vi "Configure Sweep Stimulus.vi"(4 "Signal Output (T: On)":bool=TRUE, 6 "Parameter (0.0)":dbl format="%^.2e", 7 "Channel (1)":i32=1, 8 "error in (no error)":errorcluster, 9 "Stimulus (0: Start)":u16(ring) items=["Start", "Stop", "Center", "Span"], 10 "Unit (0: Hz)":u16(ring) items=["Hz", "kHz", "MHz", "GHz", "dBm", "s", "V"], 11 "VISA resource name":refnum<visa-resource-name>) -> (0 "error out":errorcluster, 3 "VISA resource name out":refnum<visa-resource-name>)   [LabVIEW 2015, in "Agilent ENA Series.lvlib"]
doc: "This VI sets frequency, power or time sweep parameters."
uses:
  Agilent ENA Series.lvlib
panel:
  # "T: On\n\nF: Off"
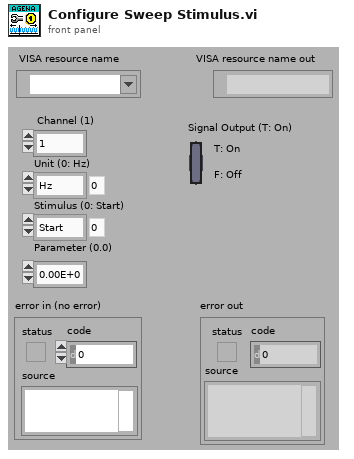
[diagram p1: front panel]
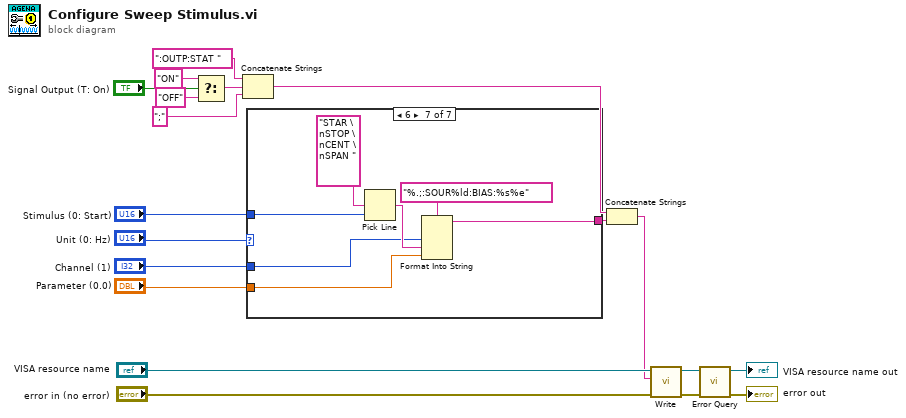
[diagram p0: block diagram]
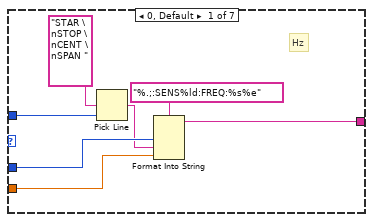
[diagram p2: hidden frame]
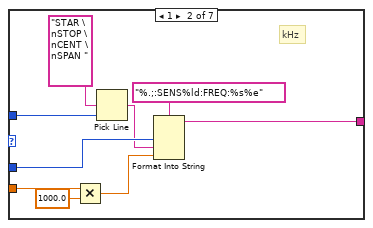
[diagram p3: hidden frame]
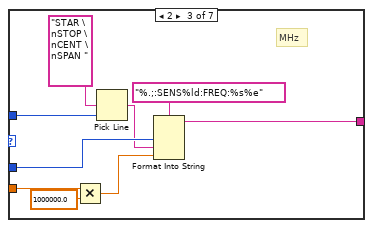
[diagram p4: hidden frame]
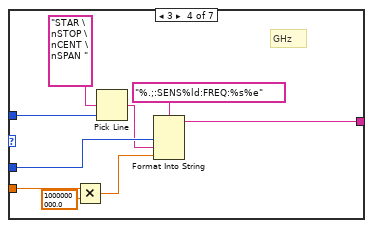
[diagram p5: hidden frame]
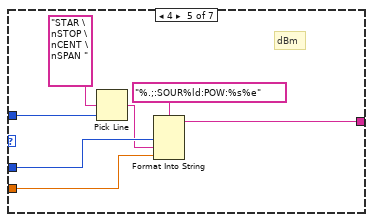
[diagram p6: hidden frame]
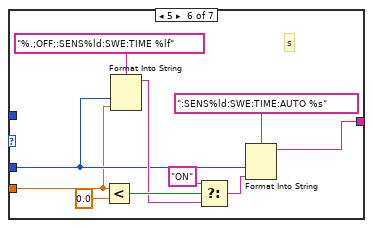
[diagram p7: hidden frame]
diagram:
  n1 = Select(t="ON", s="Signal Output (T: On)", f="OFF") -> (s? t:f=w5:string)
  n2 = Concatenate Strings(":OUTP:STAT ", w5, ";") -> (w2:string)
  n3 = case shown="6" "Unit (0: Hz)" {
    tunnel: "Parameter (0.0)" -> [w21 w30 w39 w48 w55 w63 w72]
    tunnel: "Channel (1)" -> [w25 w34 w43 w52 w59 w64 w73]
    tunnel: "Stimulus (0: Start)" -> [w22 w31 w40 w49 w56 _ w74]
    tunnel: [w20 w27 w36 w45 w54 w61 w71] -> w3
    frame 0, Default {
      # "Hz"
      n4 = Pick Line(multi-line string="STAR \nSTOP \nCENT \nSPAN ", line index=w22) -> (output string=w23:string)  [unwired: 1 in]
      n5 = Format Into String(format string="%.;:SENS%ld:FREQ:%s%e", w25, w23, w21) -> (resulting string=w20:string)  [unwired: 2 in, 1 out]
    }
    frame 1 {
      # "kHz"
      n6 = Multiply(x=w30, y=1000.0) -> (x*y=w28:dbl)
      n7 = Pick Line(multi-line string="STAR \nSTOP \nCENT \nSPAN ", line index=w31) -> (output string=w32:string)  [unwired: 1 in]
      n8 = Format Into String(format string="%.;:SENS%ld:FREQ:%s%e", w34, w32, w28) -> (resulting string=w27:string)  [unwired: 2 in, 1 out]
    }
    frame 2 {
      # "MHz"
      n9 = Multiply(x=w39, y=1000000.0) -> (x*y=w37:dbl)
      n10 = Pick Line(multi-line string="STAR \nSTOP \nCENT \nSPAN ", line index=w40) -> (output string=w41:string)  [unwired: 1 in]
      n11 = Format Into String(format string="%.;:SENS%ld:FREQ:%s%e", w43, w41, w37) -> (resulting string=w36:string)  [unwired: 2 in, 1 out]
    }
    frame 3 {
      # "GHz"
      n12 = Multiply(x=w48, y=1000000000.0) -> (x*y=w46:dbl)
      n13 = Pick Line(multi-line string="STAR \nSTOP \nCENT \nSPAN ", line index=w49) -> (output string=w50:string)  [unwired: 1 in]
      n14 = Format Into String(format string="%.;:SENS%ld:FREQ:%s%e", w52, w50, w46) -> (resulting string=w45:string)  [unwired: 2 in, 1 out]
    }
    frame 4 {
      # "dBm"
      n15 = Pick Line(multi-line string="STAR \nSTOP \nCENT \nSPAN ", line index=w56) -> (output string=w57:string)  [unwired: 1 in]
      n16 = Format Into String(format string="%.;:SOUR%ld:POW:%s%e", w59, w57, w55) -> (resulting string=w54:string)  [unwired: 2 in, 1 out]
    }
    frame 5 {
      # "s"
      n17 = Less?(x=w63, y=0.0) -> (x < y?=w67:bool)
      n18 = Format Into String(format string="%.;OFF;:SENS%ld:SWE:TIME %lf", w64, w63) -> (resulting string=w65:string)  [unwired: 2 in, 1 out]
      n19 = Select(t="ON", s=w67, f=w65) -> (s? t:f=w62:string)
      n20 = Format Into String(format string=":SENS%ld:SWE:TIME:AUTO %s", w64, w62) -> (resulting string=w61:string)  [unwired: 2 in, 1 out]
    }
    frame 6 {
      n21 = Pick Line(multi-line string="STAR \nSTOP \nCENT \nSPAN ", line index=w74) -> (output string=w77:string)  [unwired: 1 in]
      n22 = Format Into String(format string="%.;:SOUR%ld:BIAS:%s%e", w73, w77, w72) -> (resulting string=w71:string)  [unwired: 2 in, 1 out]
    }
  }
  n23 = Concatenate Strings(w2, w3) -> (w1:string)
  n24 = call "Write.vi"("error in (no error)"="error in (no error)", "String ()"=w1, "VISA resource name"="VISA resource name") -> ("error out"=w12:errorcluster, "VISA resource name out"=w13:refnum<visa-resource-name>)  [unwired: 6 in, 1 out]
  n25 = call "Error Query.vi"("error in (no error)"=w12, "VISA resource name"=w13) -> ("error out"=→"error out":errorcluster, "VISA resource name out"=→"VISA resource name out":refnum<visa-resource-name>)  [unwired: 6 in, 2 out]
